vi "NI VeriStand - Close Command Line Notification (Macro Recorder).vi"(8 "error in (no error)":errorcluster, 11 "CommandLine Refs":T1) -> (0 "error out":errorcluster)   [LabVIEW 2020, in "NI_VS MacroRecorderAPI.lvlib"]
doc: "Closes an open reference to the command line of the Macro Recorder tool. Use the Open Command Line Notification (Macro Recorder) VI to open the reference this VI closes."
uses:
  <vilib>/NI VeriStand/Execution/MacroRecorder/NI_VS MacroRecorderAPI.lvlib
  <vilib>/NI VeriStand/Execution/MacroRecorder/CommandLine Refs.ctl
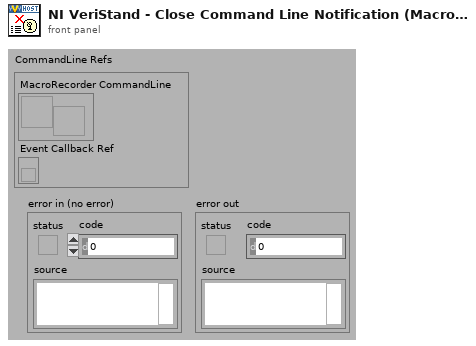
[diagram p1: front panel]
types:
  T1 = typedef "NI_VS MacroRecorderAPI.lvlib/CommandLine Refs.ctl" = cluster{"MacroRecorder CommandLine":refnum<user-event>, "Event Callback Ref":refnum<k27>}
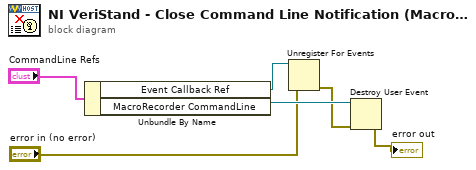
[diagram p0: block diagram]
diagram:
  n1 = Unbundle By Name("CommandLine Refs") -> ("Event Callback Ref"=w5:refnum<k27>, "MacroRecorder CommandLine"=w4:refnum<user-event>)
  n2 = Unregister For Events(event registration refnum=w5, error in="error in (no error)") -> (error out=w3:errorcluster)
  n3 = Destroy User Event(user event=w4, error in=w3) -> (error out=→"error out":errorcluster)
